vi "NHR-5200.vi"() -> ()   [LabVIEW 2018]
uses:
  <vilib>/Modbus/master/Create Master Instance (Serial).vi
  <vilib>/Modbus/master/Modbus Master.lvclass
panel:
  in  "?":string
  in  "?":string
  in  "?":string
  out "register values":u16[](array[numeric]) caption="Value"
  in  "?":bool
  in  "holding register value":u16 caption="Value"
  in  "address":u16 caption="WriteAddr"
  in  "number of holding registers":u16 caption="Length"
  in  "starting address":u16 caption="ReadAddr"
  in  "SerialPort":refnum<visa-resource-name>
  in  "serial type":enum16{"RTU", "ASCII"}(ring)
  in  "BaudRate":u32=9600
  in  "Device ID":u8=1
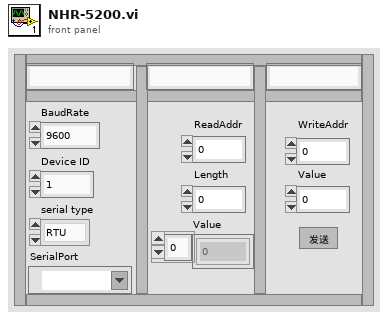
[diagram p1: front panel]
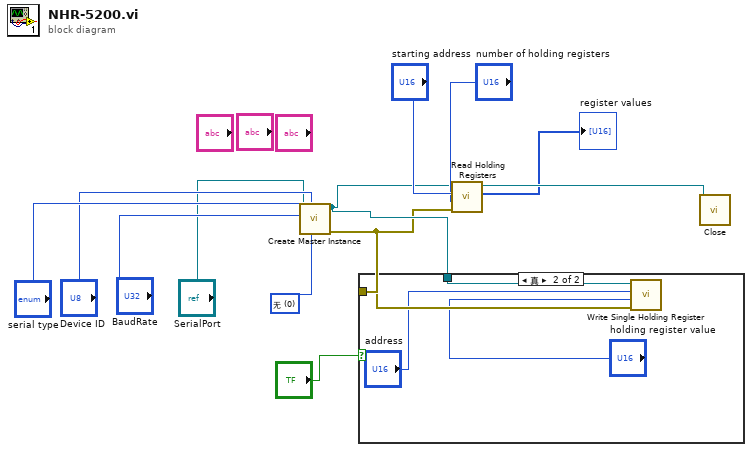
[diagram p0: block diagram]
diagram:
  w11 = u16 0 items=["无", "奇", "偶"] ("parity (Even)")
  n1 = call-poly <vilib>:"Create Master Instance.vi"("serial type"="serial type", "parity (Even)"=w11, "unit ID"="Device ID", "baud rate (9600)"="BaudRate", "VISA resource name"="SerialPort") -> ("error out"=w3:errorcluster, "serial master instance"=w4:refnum<class "Modbus Master.lvclass">)  [unwired: 5 in]
  n2 = case shown="真" "?" {
    tunnel: w4 -> [_ w16]
    tunnel: w3 -> [_ w15]
    frame False {
    }
    frame True {
      n3 = call-dynamic "Write Single Holding Register.vi"("error in (no error)"=w15, "holding register value"="holding register value", "address"="address", "Modbus master in"=w16) -> ()  [unwired: 6 in, 2 out]
    }
  }
  n4 = call-dynamic "Read Holding Registers.vi"("error in (no error)"=w3, "number of holding registers"="number of holding registers", "starting address"="starting address", "Modbus master in"=w4) -> ("register values"=→"register values":u16[], "Modbus master out"=w5:refnum<class "Modbus Master.lvclass">)  [unwired: 5 in, 1 out]
  n5 = call-dynamic "Close.vi"("Modbus master in"=w5) -> ()  [unwired: 10 in, 1 out]
